vi "Subtract Dates.vi"(8 "error in (no error)":errorcluster, 10 "First date":string="25/09/2005", 11 "Second date":string="25/09/2006") -> (0 "error out":errorcluster, 3 "Elapsed days":i32)   [LabVIEW 2022 SP3]
doc: "This VI outputs the number of elapsed days between two specified date strings. The VI converts the date strings to timestamps. It then uses those timestamps to calculate the number of elapsed days between the two dates."
panel:
  out "x-y*floor(x/y)":i32
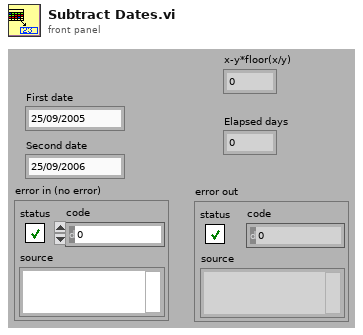
[diagram p1: front panel]
types:
  T1 = cluster{"fractional second":dbl, "second":i32, "minute":i32, "hour":i32, "day of month":i32, "month":i32, "year":i32, "day of week":i32, "day of year":i32, "DST":i32}
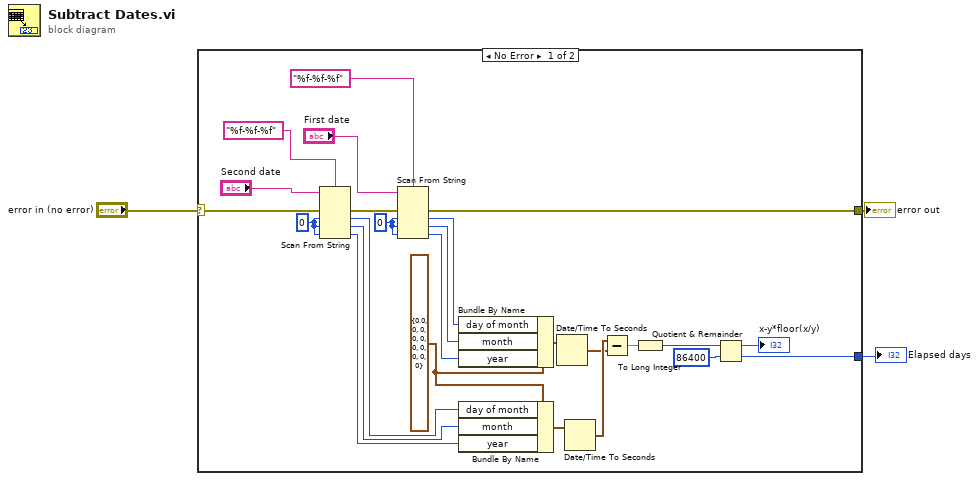
[diagram p0: block diagram]
diagram:
  n1 = case shown="No Error" "error in (no error)" {
    selector: "error in (no error)" -> [w10 w29]
    tunnel: [w11 w29] -> w2
    tunnel: [w7 _] -> w1
    frame No Error {
      w15 = T1 {"fractional second"=0.0, "second"=0, "minute"=0, "hour"=0, "day of month"=0, "month"=0, "year"=0, "day of week"=0, "day of year"=0, "DST"=0} ("date time rec")
      w26 = 0
      w27 = 0
      n2 = Scan From String(format string="%f-%f-%f", input string="Second date", error in=w10, default 1=w27, default 2=w27, default 3=w27) -> (error out=w12:errorcluster, output 1=w22:i32, output 2=w21:i32, output 3=w20:i32)  [unwired: 1 in, 2 out]
      n3 = Scan From String(format string="%f-%f-%f", input string="First date", error in=w12, default 1=w26, default 2=w26, default 3=w26) -> (error out=w11:errorcluster, output 1=w19:i32, output 2=w18:i32, output 3=w17:i32)  [unwired: 1 in, 2 out]
      n4 = Bundle By Name(cluster=w15, "day of month"=w19, "month"=w18, "year"=w17) -> (w23:T1)
      n5 = Bundle By Name(cluster=w15, "day of month"=w22, "month"=w21, "year"=w20) -> (w24:T1)
      n6 = Date/Time To Seconds(2:w23) -> (0:w4:timestamp)  [unwired: 1 in]
      n7 = Date/Time To Seconds(2:w24) -> (0:w5:timestamp)  [unwired: 1 in]
      n8 = Subtract(x=w5, y=w4) -> (x-y=w16:dbl)
      n9 = To Long Integer(number=w16) -> (32bit integer=w13:i32)
      n10 = Quotient & Remainder(x=w13, y=86400) -> (x-y*floor(x/y)=→"x-y*floor(x/y)":i32, floor(x/y)=w7:i32)
    }
    frame Error {
    }
  }
  "error out" <- w2
  "Elapsed days" <- w1
